vi "Generic command handler.vi"(8 "error in (no error)":errorcluster, 10 "Message in":refnum<class "GenericMessage.lvclass">, 11 "Thorcam in":refnum<class "Thorcam.lvclass">) -> (0 "error out":errorcluster, 2 "value":string, 3 "Thorcam out":refnum<class "Thorcam.lvclass">)   [LabVIEW 2012, in "Thorcam.lvclass"]
doc: "The generic_command_handler processes the command 'generic'. Commands which are not part of the predefined list of commands fall under the 'generic' command for special activity."
uses:
  Thorcam.lvclass
  <vilib>/Distrio/Murmex/GenericMessage/GenericMessage.lvclass
  <vilib>/Distrio/Murmex/Murmex/Murmex.lvclass
  <vilib>/Distrio/Murmex/ProceedMessage/ProceedMessage.lvclass
  Thorcam.lvclass/Thorcam.ctl
  current task.ctl
  <vilib>/vision/NI_Vision_Development_Module.lvlib
panel:
  # "This method is called when the GENERIC\ntrigger is sent. \n\nOverride this method when your component needs to\nrespond to this trigger. \n\nCall parent for proper implementation"
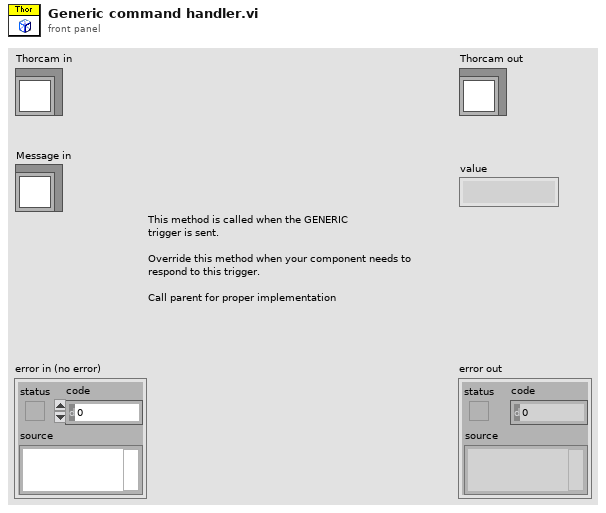
[diagram p1: front panel]
types:
  T1 = typedef "Thorcam.lvclass/current task.ctl" = enum16{"Camera", "Phase Comparison", "Pre-Tomo"}
  T2 = typedef "Thorcam.lvclass/feed.ctl" = enum16{"Video", "Cross Correlation", "Rob and Roy", "Roy", "Rob"}
  T3 = typedef "IMAQ Image.ctl" = refnum<image>
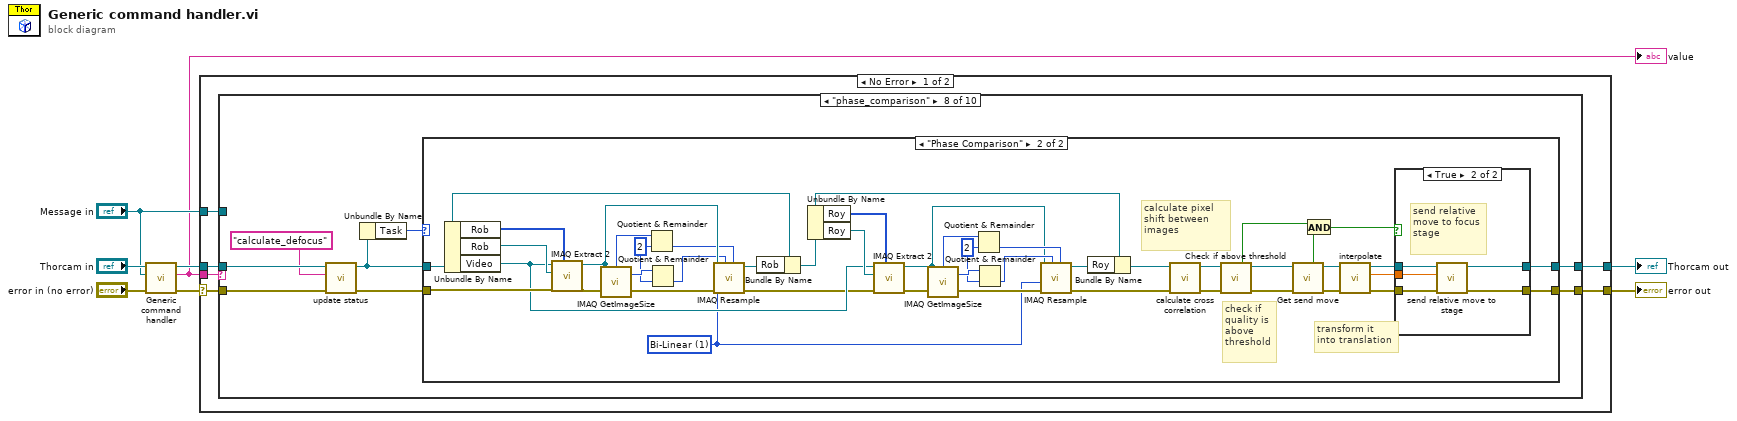
[diagram p0: block diagram]
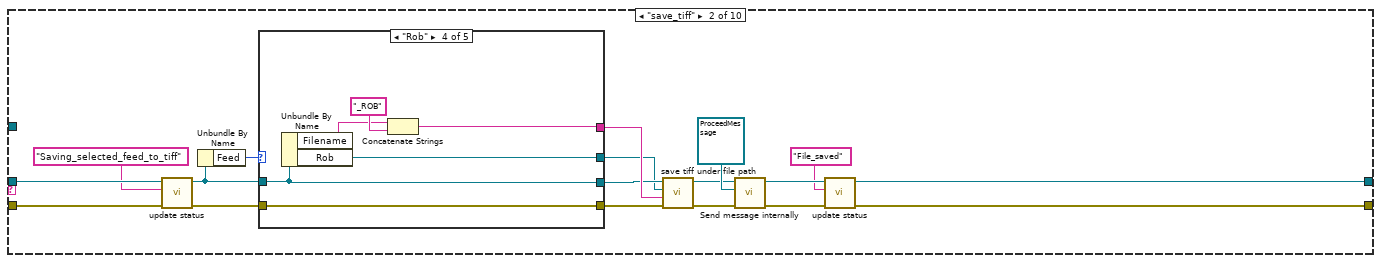
[diagram p3: hidden frame]
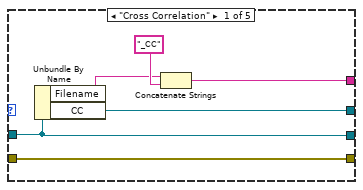
[diagram p4: hidden frame]
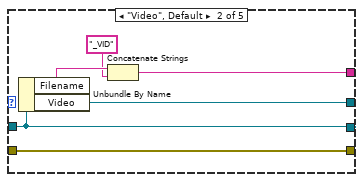
[diagram p5: hidden frame]
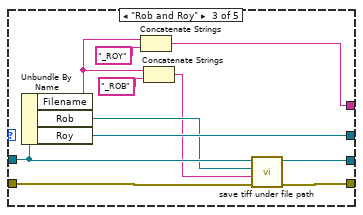
[diagram p6: hidden frame]
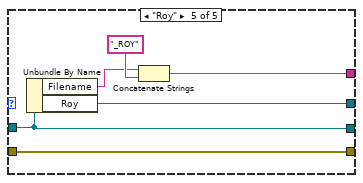
[diagram p7: hidden frame]
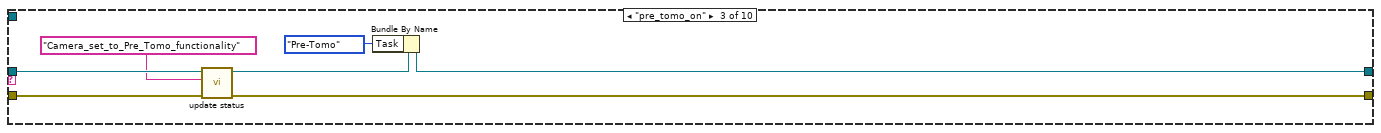
[diagram p8: hidden frame]
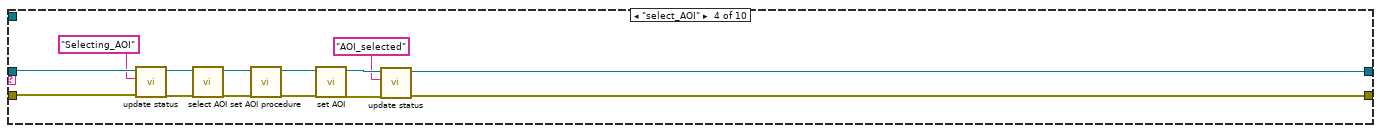
[diagram p9: hidden frame]
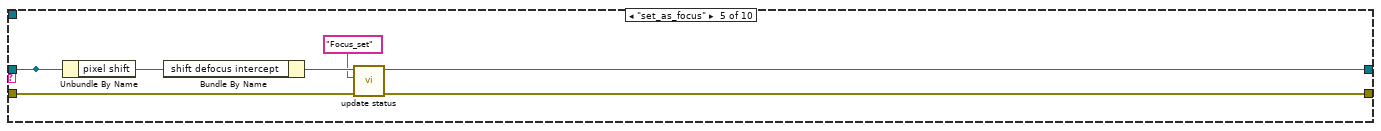
[diagram p10: hidden frame]
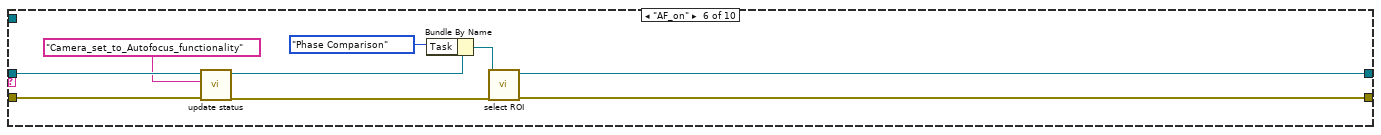
[diagram p11: hidden frame]
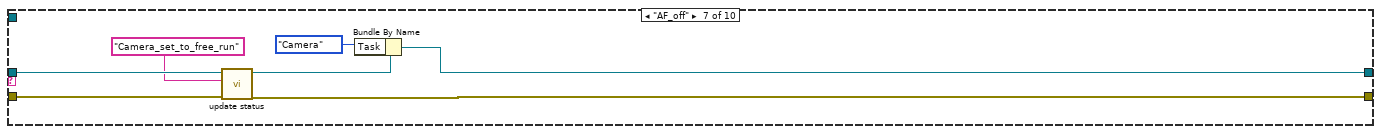
[diagram p12: hidden frame]
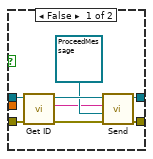
[diagram p14: hidden frame]
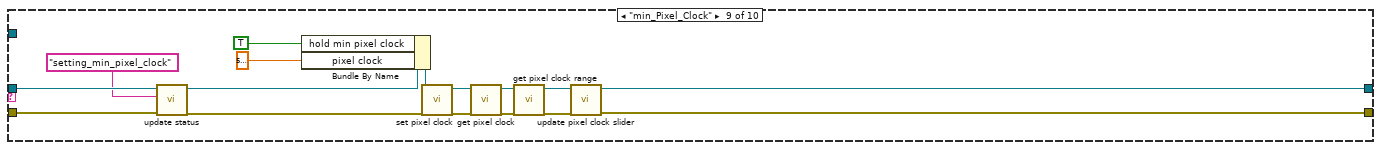
[diagram p15: hidden frame]
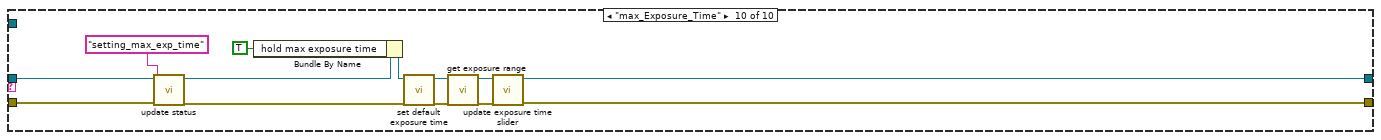
[diagram p16: hidden frame]
diagram:
  n1 = call-parent "Generic command handler.vi"("error in (no error)"="error in (no error)", "Message in"="Message in", "Murmex in"="Thorcam in") -> ("error out"=w6:errorcluster, "value"=w3:string, "Murmex out"=w5:refnum<class "Thorcam.lvclass">)  [unwired: 6 in]
  "value" <- w3
  n2 = case shown="No Error" w6 {
    selector: w6 -> [w14 w210]
    tunnel: w3 -> [w13 _]
    tunnel: w5 -> [w12 w211]
    tunnel: "Message in" -> [w11 _]
    tunnel: [w10 w210] -> w2
    tunnel: [w9 w211] -> w1
    frame No Error {
      n3 = case shown="\"phase_comparison\"" w13 {
        tunnel: w14 -> [w15 w27 w74 w90 w95 w102 w112 w119 w185 w202]
        tunnel: w12 -> [w16 w25 w72 w88 w97 w100 w111 w117 w183 w198]
        tunnel: w11 -> [_ _ _ _ _ _ _ _ _ _]
        tunnel: [w15 w20 w73 w80 w94 w103 w107 w114 w187 w203] -> w10
        tunnel: [w16 w18 w75 w78 w92 w104 w108 w121 w188 w204] -> w9
        frame Default {
        }
        frame "save_tiff" {
          n4 = call-dynamic "update status.vi"("error in (no error)"=w27, "status in"="Saving_selected_feed_to_tiff", "Thorcam in"=w25) -> ("error out"=w26:errorcluster, "Thorcam out"=w24:refnum<class "Thorcam.lvclass">)  [unwired: 7 in]
          n5 = Unbundle By Name(w24) -> ("Feed"=w32:T2)
          n6 = case shown="\"Rob\"" w32 {
            tunnel: w26 -> [w40 w43 w50 w63 w69]
            tunnel: [w40 w43 w52 w63 w69] -> w30
            tunnel: w24 -> [w39 w42 w49 w62 w68]
            tunnel: [w39 w42 w51 w62 w68] -> w29
            tunnel: [w38 w41 w57 w61 w67] -> w28
            tunnel: [w36 w44 w55 w59 w65] -> w31
            frame "Cross Correlation" {
              n7 = Unbundle By Name(w39) -> ("Filename"=w35:string, "CC"=w38:T3)
              n8 = Concatenate Strings(w35, "_CC" ("string")) -> (w36:string)
            }
            frame "Video", Default {
              n9 = Unbundle By Name(w42) -> ("Filename"=w46:string, "Video"=w41:T3)
              n10 = Concatenate Strings(w46, "_VID" ("string")) -> (w44:string)
            }
            frame "Rob and Roy" {
              n11 = Unbundle By Name(w49) -> ("Filename"=w53:string, "Rob"=w48:T3, "Roy"=w57:T3)
              n12 = Concatenate Strings(w53, "_ROY" ("string")) -> (w55:string)
              n13 = Concatenate Strings(w53, "_ROB" ("string")) -> (w47:string)
              n14 = call-dynamic "save tiff under file path.vi"("error in (no error)"=w50, "tiff name"=w47, "Image"=w48, "Thorcam in"=w49) -> ("error out"=w52:errorcluster, "Thorcam out"=w51:refnum<class "Thorcam.lvclass">)  [unwired: 6 in]
            }
            frame "Rob" {
              n15 = Unbundle By Name(w62) -> ("Filename"=w58:string, "Rob"=w61:T3)
              n16 = Concatenate Strings(w58, "_ROB" ("string")) -> (w59:string)
            }
            frame "Roy" {
              n17 = Unbundle By Name(w68) -> ("Filename"=w64:string, "Roy"=w67:T3)
              n18 = Concatenate Strings(w64, "_ROY" ("string")) -> (w65:string)
            }
          }
          n19 = call-dynamic "save tiff under file path.vi"("error in (no error)"=w30, "tiff name"=w31, "Image"=w28, "Thorcam in"=w29) -> ("error out"=w33:errorcluster, "Thorcam out"=w22:refnum<class "Thorcam.lvclass">)  [unwired: 6 in]
          n20 = call <vilib>:"Send message internally.vi"("error in (no error)"=w33, "Message"=refnum<class "ProceedMessage.lvclass"> refnum ("Distrio Murmex 1.5:ProceedMessage"), "Murmex in"=w22) -> ("error out"=w21:errorcluster, "Murmex out"=w19:refnum<class "Thorcam.lvclass">)  [unwired: 7 in]
          n21 = call-dynamic "update status.vi"("error in (no error)"=w21, "status in"="File_saved", "Thorcam in"=w19) -> ("error out"=w20:errorcluster, "Thorcam out"=w18:refnum<class "Thorcam.lvclass">)  [unwired: 7 in]
        }
        frame "pre_tomo_on" {
          n22 = call-dynamic "update status.vi"("error in (no error)"=w74, "status in"="Camera_set_to_Pre_Tomo_functionality", "Thorcam in"=w72) -> ("error out"=w73:errorcluster, "Thorcam out"=w71:refnum<class "Thorcam.lvclass">)  [unwired: 7 in]
          n23 = Bundle By Name(cluster=w71, "Task"=current_task."Pre-Tomo" ("runtime.Task")) -> (w75:refnum<class "Thorcam.lvclass">)
        }
        frame "select_AOI" {
          n24 = call-dynamic "update status.vi"("error in (no error)"=w90, "status in"="Selecting_AOI", "Thorcam in"=w88) -> ("error out"=w89:errorcluster, "Thorcam out"=w86:refnum<class "Thorcam.lvclass">)  [unwired: 7 in]
          n25 = call-dynamic "select AOI.vi"("error in (no error)"=w89, "Thorcam in"=w86) -> ("error out"=w85:errorcluster, "Thorcam out"=w84:refnum<class "Thorcam.lvclass">)  [unwired: 8 in]
          n26 = call-dynamic "set AOI procedure.vi"("error in (no error)"=w85, "Thorcam in"=w84) -> ("error out"=w83:errorcluster, "Thorcam out"=w82:refnum<class "Thorcam.lvclass">)  [unwired: 8 in]
          n27 = call-dynamic "set AOI.vi"("error in (no error)"=w83, "Thorcam in"=w82) -> ("error out"=w81:errorcluster, "Thorcam out"=w79:refnum<class "Thorcam.lvclass">)  [unwired: 8 in]
          n28 = call-dynamic "update status.vi"("error in (no error)"=w81, "status in"="AOI_selected", "Thorcam in"=w79) -> ("error out"=w80:errorcluster, "Thorcam out"=w78:refnum<class "Thorcam.lvclass">)  [unwired: 7 in]
        }
        frame "set_as_focus" {
          n29 = Unbundle By Name(w97) -> ("pixel shift"=w96:dbl)
          n30 = Bundle By Name(cluster=w97, "shift defocus intercept"=w96) -> (w93:refnum<class "Thorcam.lvclass">)
          n31 = call-dynamic "update status.vi"("error in (no error)"=w95, "status in"="Focus_set", "Thorcam in"=w93) -> ("error out"=w94:errorcluster, "Thorcam out"=w92:refnum<class "Thorcam.lvclass">)  [unwired: 7 in]
        }
        frame "AF_on" {
          n32 = call-dynamic "update status.vi"("error in (no error)"=w102, "status in"="Camera_set_to_Autofocus_functionality", "Thorcam in"=w100) -> ("error out"=w101:errorcluster, "Thorcam out"=w99:refnum<class "Thorcam.lvclass">)  [unwired: 7 in]
          n33 = Bundle By Name(cluster=w99, "Task"=current_task."Phase Comparison" ("runtime.Task")) -> (w105:refnum<class "Thorcam.lvclass">)
          n34 = call-dynamic "select ROI.vi"("error in (no error)"=w101, "Thorcam in"=w105) -> ("error out"=w103:errorcluster, "Thorcam out"=w104:refnum<class "Thorcam.lvclass">)  [unwired: 8 in]
        }
        frame "AF_off" {
          n35 = call-dynamic "update status.vi"("error in (no error)"=w112, "status in"="Camera_set_to_free_run", "Thorcam in"=w111) -> ("error out"=w107:errorcluster, "Thorcam out"=w110:refnum<class "Thorcam.lvclass">)  [unwired: 7 in]
          n36 = Bundle By Name(cluster=w110, "Task"=current_task."Camera" ("runtime.Task")) -> (w108:refnum<class "Thorcam.lvclass">)
        }
        frame "phase_comparison" {
          n37 = call-dynamic "update status.vi"("error in (no error)"=w119, "status in"="calculate_defocus", "Thorcam in"=w117) -> ("error out"=w118:errorcluster, "Thorcam out"=w116:refnum<class "Thorcam.lvclass">)  [unwired: 7 in]
          n38 = Unbundle By Name(w116) -> ("Task"=w120:T1)
          n39 = case shown="\"Phase Comparison\"" w120 {
            tunnel: w118 -> [w122 w155]
            tunnel: [w122 w157] -> w114
            tunnel: [w123 w158] -> w121
            tunnel: w116 -> [w123 w156]
            frame "Camera", Default {
            }
            frame "Phase Comparison" {
              w124 = u32 1 items=["Zero Order", "Bi-Linear", "Quadratic", "Cubic Spline"] ("Interpolation Type")
              w131 = 2 ("y")
              w137 = 2 ("y")
              # "check if\nquality is\nabove\nthreshold"
              # "calculate pixel\nshift between\nimages"
              # "transform it\ninto translation"
              n40 = Unbundle By Name(w156) -> ("Rob"=w166:i32[], "Rob"=w167:T3, "Video"=w154:T3)
              n41 = call "IMAQ Extract 2"("Optional Rectangle"=w166, "error in (no error)"=w155, "Image Dst"=w167, "Image Src"=w154) -> ("error out"=w143:errorcluster, "Image Dst Out"=w141:T3)  [unwired: 6 in]
              n42 = call "IMAQ GetImageSize"("Image"=w141, "error in (no error)"=w143) -> ("Y Resolution"=w138:i32, "X Resolution"=w139:i32, "error out"=w144:errorcluster)  [unwired: 2 in]
              n43 = Quotient & Remainder(x=w139, y=w137) -> (floor(x/y)=w135:i32)  [unwired: 1 out]
              n44 = Quotient & Remainder(x=w138, y=w137) -> (floor(x/y)=w136:i32)  [unwired: 1 out]
              n45 = call "IMAQ Resample"("X Resolution"=w135, "Y Resolution"=w136, "error in (no error)"=w144, "Interpolation Type"=w124, "Image Src"=w141) -> ("error out"=w142:errorcluster, "Image Dst Out"=w140:T3)  [unwired: 5 in]
              n46 = Bundle By Name(cluster=w156, "Rob"=w140) -> (w163:refnum<class "Thorcam.lvclass">)
              n47 = Unbundle By Name(w163) -> ("Roy"=w165:i32[], "Roy"=w164:T3)
              n48 = call "IMAQ Extract 2"("Optional Rectangle"=w165, "error in (no error)"=w142, "Image Dst"=w164, "Image Src"=w154) -> ("error out"=w128:errorcluster, "Image Dst Out"=w126:T3)  [unwired: 6 in]
              n49 = call "IMAQ GetImageSize"("Image"=w126, "error in (no error)"=w128) -> ("Y Resolution"=w132:i32, "X Resolution"=w133:i32, "error out"=w134:errorcluster)  [unwired: 2 in]
              n50 = Quotient & Remainder(x=w133, y=w131) -> (floor(x/y)=w129:i32)  [unwired: 1 out]
              n51 = Quotient & Remainder(x=w132, y=w131) -> (floor(x/y)=w130:i32)  [unwired: 1 out]
              n52 = call "IMAQ Resample"("X Resolution"=w129, "Y Resolution"=w130, "error in (no error)"=w134, "Interpolation Type"=w124, "Image Src"=w126) -> ("error out"=w127:errorcluster, "Image Dst Out"=w125:T3)  [unwired: 5 in]
              n53 = Bundle By Name(cluster=w163, "Roy"=w125) -> (w159:refnum<class "Thorcam.lvclass">)
              n54 = call-dynamic "calculate cross correlation.vi"("error in (no error)"=w127, "Thorcam in"=w159) -> ("error out"=w152:errorcluster, "Thorcam out"=w153:refnum<class "Thorcam.lvclass">)  [unwired: 8 in]
              n55 = call-dynamic "Check if above threshold.vi"("error in (no error)"=w152, "Thorcam in"=w153) -> ("error out"=w149:errorcluster, "above threshold?"=w147:bool, "Thorcam out"=w151:refnum<class "Thorcam.lvclass">)  [unwired: 7 in]
              n56 = call-dynamic "Get send move.vi"("error in (no error)"=w149, "Thorcam in"=w151) -> ("error out"=w148:errorcluster, "Send move?"=w145:bool, "Thorcam out"=w150:refnum<class "Thorcam.lvclass">)  [unwired: 7 in]
              n57 = And(x=w147, y=w145) -> (x .and. y?=w146:bool)
              n58 = call-dynamic "interpolate.vi"("error in (no error)"=w148, "Thorcam in"=w150) -> ("error out"=w162:errorcluster, "position out"=w160:dbl[unit], "Thorcam out"=w161:refnum<class "Thorcam.lvclass">)  [unwired: 7 in]
              n59 = case shown="True" w146 {
                tunnel: w162 -> [w174 w180]
                tunnel: w161 -> [w175 w179]
                tunnel: w160 -> [_ w178]
                tunnel: [w170 w177] -> w158
                tunnel: [w169 w176] -> w157
                frame False {
                  n60 = call <vilib>:"Get ID.vi"("error in (no error)"=w174, "Murmex in"=w175) -> ("error out"=w171:errorcluster, "component id"=w168:string, "Murmex out"=w173:refnum<class "Thorcam.lvclass">)  [unwired: 7 in]
                  n61 = call <vilib>:"Send.vi"("error in (no error)"=w171, "Message"=refnum<class "ProceedMessage.lvclass"> refnum ("Distrio Murmex 1.5:ProceedMessage"), "recipient"=w168, "Murmex in"=w173) -> ("error out"=w169:errorcluster, "Murmex out"=w170:refnum<class "Thorcam.lvclass">)  [unwired: 6 in]
                }
                frame True {
                  # "send relative move to focus stage"
                  n62 = call-dynamic "send relative move to stage.vi"("error in (no error)"=w180, "relative move to send"=w178, "Thorcam in"=w179) -> ("error out"=w176:errorcluster, "Thorcam out"=w177:refnum<class "Thorcam.lvclass">)  [unwired: 7 in]
                }
              }
            }
          }
        }
        frame "min_Pixel_Clock" {
          n63 = call-dynamic "update status.vi"("error in (no error)"=w185, "status in"="setting_min_pixel_clock", "Thorcam in"=w183) -> ("error out"=w184:errorcluster, "Thorcam out"=w182:refnum<class "Thorcam.lvclass">)  [unwired: 7 in]
          n64 = Bundle By Name(cluster=w182, "hold min pixel clock"=TRUE ("runtime.pixel clock range.hold minimum"), "pixel clock"=dbl[unit] 5000000.0 ("settings.Camera settings.pixel clock")) -> (w196:refnum<class "Thorcam.lvclass">)
          n65 = call-dynamic "set pixel clock.vi"("error in (no error)"=w184, "Thorcam in"=w196) -> ("error out"=w193:errorcluster, "Thorcam out"=w194:refnum<class "Thorcam.lvclass">)  [unwired: 8 in]
          n66 = call-dynamic "get pixel clock.vi"("error in (no error)"=w193, "Thorcam in"=w194) -> ("error out"=w191:errorcluster, "Thorcam out"=w192:refnum<class "Thorcam.lvclass">)  [unwired: 8 in]
          n67 = call-dynamic "get pixel clock range.vi"("error in (no error)"=w191, "Thorcam in"=w192) -> ("error out"=w189:errorcluster, "Thorcam out"=w190:refnum<class "Thorcam.lvclass">)  [unwired: 8 in]
          n68 = call-dynamic "update pixel clock slider.vi"("error in (no error)"=w189, "Thorcam in"=w190) -> ("error out"=w187:errorcluster, "Thorcam out"=w188:refnum<class "Thorcam.lvclass">)  [unwired: 8 in]
        }
        frame "max_Exposure_Time" {
          n69 = call-dynamic "update status.vi"("error in (no error)"=w202, "status in"="setting_max_exp_time", "Thorcam in"=w198) -> ("error out"=w201:errorcluster, "Thorcam out"=w200:refnum<class "Thorcam.lvclass">)  [unwired: 7 in]
          n70 = Bundle By Name(cluster=w200, "hold max exposure time"=TRUE ("runtime.pixel clock range.hold minimum")) -> (w199:refnum<class "Thorcam.lvclass">)
          n71 = call-dynamic "set default exposure time.vi"("error in (no error)"=w201, "Thorcam in"=w199) -> ("error out"=w208:errorcluster, "Thorcam out"=w207:refnum<class "Thorcam.lvclass">)  [unwired: 7 in, 1 out]
          n72 = call-dynamic "get exposure range.vi"("error in (no error)"=w208, "Thorcam in"=w207) -> ("error out"=w205:errorcluster, "Thorcam out"=w206:refnum<class "Thorcam.lvclass">)  [unwired: 8 in]
          n73 = call-dynamic "update exposure time slider.vi"("error in (no error)"=w205, "Thorcam in"=w206) -> ("error out"=w203:errorcluster, "Thorcam out"=w204:refnum<class "Thorcam.lvclass">)  [unwired: 8 in]
        }
      }
    }
    frame Error {
    }
  }
  "error out" <- w2
  "Thorcam out" <- w1
